vi "Save Notebook Rich Text Box.vi"(6 "Backup?":bool, 7 "Default Notebook File Name (Notebook)":string="Notebook", 8 "Error In":errorcluster, 9 "Dialog (F)":bool, 10 "File Path Control":path, 11 ".NET Refnum in":refnum<k24>) -> (0 "Error Out":errorcluster, 1 "cancelled":bool, 2 "File Path out":path)   [LabVIEW 2019, in "Notebook.lvlib"]
uses:
  Notebook.lvlib
  System.Windows.Forms
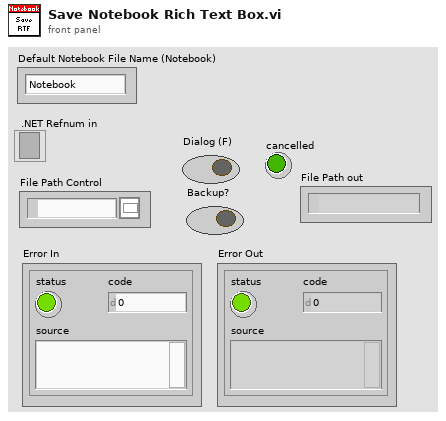
[diagram p1: front panel]
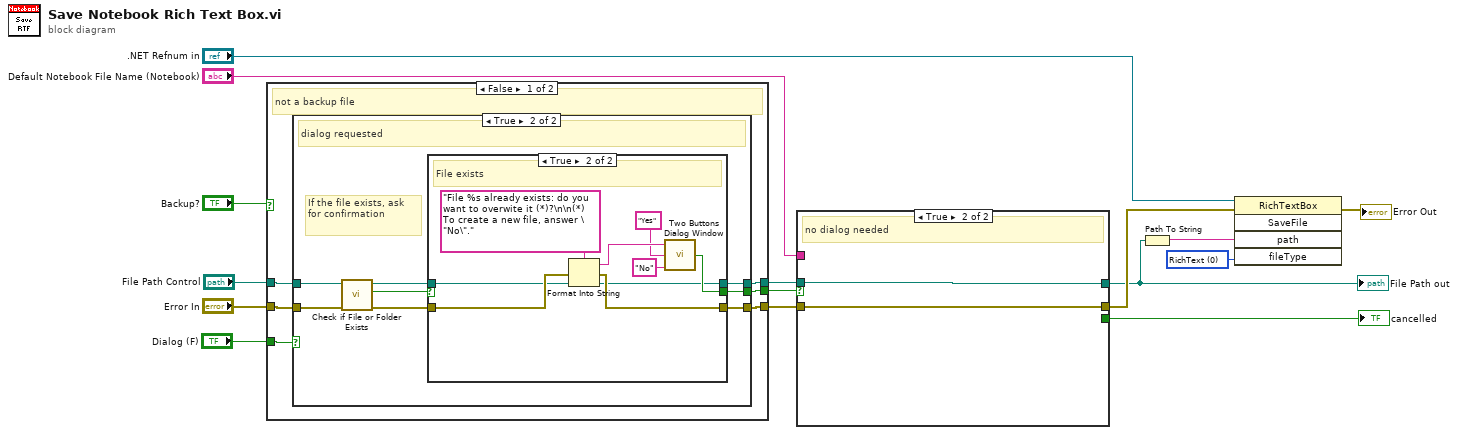
[diagram p0: block diagram]
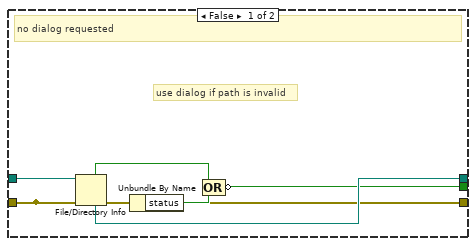
[diagram p2: hidden frame]
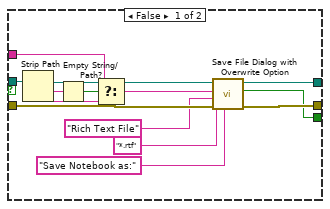
[diagram p5: hidden frame]
diagram:
  w10 = 0 items=["RichText", "PlainText", "RichNoOleObjs", "TextTextOleObjs", "UnicodePlainText"] ("fileType")
  n1 = case shown="False" "Backup?" {
    selector: "Backup?" -> [_ w50]
    tunnel: [w19 w49] -> w8
    tunnel: [w21 w48] -> w7
    tunnel: [w20 w50] -> w6
    tunnel: "Dialog (F)" -> [w16 _]
    tunnel: "File Path Control" -> [w18 w49]
    tunnel: "Error In" -> [w17 w48]
    frame False {
      # "not a backup file"
      n2 = case shown="True" w16 {
        tunnel: [w22 w36] -> w21
        tunnel: [w23 w35] -> w20
        tunnel: [w27 w34] -> w19
        tunnel: w18 -> [w28 w33]
        tunnel: w17 -> [w22 w32]
        frame False {
          # "use dialog if path is invalid"
          # "no dialog requested"
          n3 = File/Directory Info(path=w28, error in=w22) -> (directory=w24:bool, error out=w26:errorcluster, resolved path=w27:path)  [unwired: 4 out]
          n4 = Unbundle By Name(w26) -> ("status"=w25:bool)
          n5 = Compound Arithmetic op=OR(w24, w25) -> (invert w23:bool)
        }
        frame True {
          # "If the file exists, ask for confirmation"
          # "dialog requested"
          n6 = call <vilib>:"Check if File or Folder Exists.vi"("error in (no error)"=w32, "path"=w33) -> ("error out"=w31:errorcluster, "file or folder exists?"=w29:bool, "dup path"=w30:path)  [unwired: 7 in]
          n7 = case shown="True" w29 {
            selector: w29 -> [w37 _]
            tunnel: w31 -> [w38 w45]
            tunnel: [w38 w44] -> w36
            tunnel: [w37 w41] -> w35
            tunnel: w30 -> [w39 w40]
            tunnel: [w39 w40] -> w34
            frame False {
              # "File does not exist"
            }
            frame True {
              # "File exists"
              n8 = Format Into String(format string="File %s already exists: do you want to overwite it (*)?\n\n(*) To create a new file, answer \"No\".", error in=w45, w40) -> (resulting string=w46:string, error out=w44:errorcluster)  [unwired: 1 in]
              n9 = call "Two Buttons Dialog Window.vi"("Cancel Button Text"="No" ("F button name (\"Cancel\")"), "OK Button Text"="Yes" ("T button name (\"OK\")"), "Message"=w46) -> ("OK?"=w41:bool)
            }
          }
        }
      }
    }
    frame True {
      # "backup: no dialog"
    }
  }
  n10 = case shown="True" w6 {
    tunnel: [w62 w64] -> w12
    tunnel: [w61 w65] -> w14
    tunnel: w8 -> [w60 w64]
    tunnel: w7 -> [w59 w65]
    tunnel: [w57 _] -> w11
    tunnel: "Default Notebook File Name (Notebook)" -> [w51 _]
    frame False {
      n11 = Strip Path(path=w60) -> (stripped path=w58:path, name=w52:string)
      n12 = Empty String/Path?(string/path=w52) -> (empty?=w54:bool)
      n13 = Select(t=w51, s=w54, f=w52) -> (s? t:f=w53:string)
      n14 = call "Save File Dialog with Overwrite Option.vi"("prompt"="Save Notebook as:", "Default Name"=w53, "error in (no error)"=w59, "pattern label"="Rich Text File", "pattern (all files)"="*.rtf" ("pattern label"), "Starting Folder"=w58) -> ("error out"=w61:errorcluster, "cancelled"=w57:bool, "selected path"=w62:path)  [unwired: 2 in, 1 out]
    }
    frame True {
      # "no dialog needed"
    }
  }
  "File Path out" <- w12
  "cancelled" <- w11
  n15 = Path To String(path=w12) -> (string=w9:string)
  n16 = invoke class="RichTextBox" method="SaveFile"(reference=".NET Refnum in", error in=w14, "path"=w9, "fileType"=w10) -> (error out=→"Error Out":errorcluster)  [unwired: 1 in, 4 out]
